vi "FIR_5decimate_5cycles.vi"(7 "reset":bool, 8 "valid in":bool, 10 "Q in":fxp<+/-,16,14>, 11 "I in":fxp<+/-,16,14>) -> (0 "valid out":bool, 2 "Q out":fxp<+/-,16,14>, 3 "I out":fxp<+/-,16,14>, 4 "ready for input":bool)   [LabVIEW 2013]
uses:
  <vilib>/rvi/IPIntegrationNode/IPINode_Utilities/niFpgaIPINodeSimCore.vi
  <vilib>/rvi/XilinxIP/XIPIN_XNode/niFpgaXIPIN.xnode
  Filters/FIR_5decimate_5cycles/FIR_5Decimate_5Cycles_B5291933BF2B454885F1E12D573C96C6.dll
  <vilib>/rvi/IPIntegrationNode/IPINode_Xnode/niFpgaIPINode.xnode
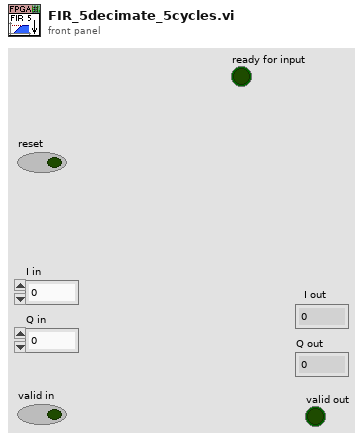
[diagram p1: front panel]
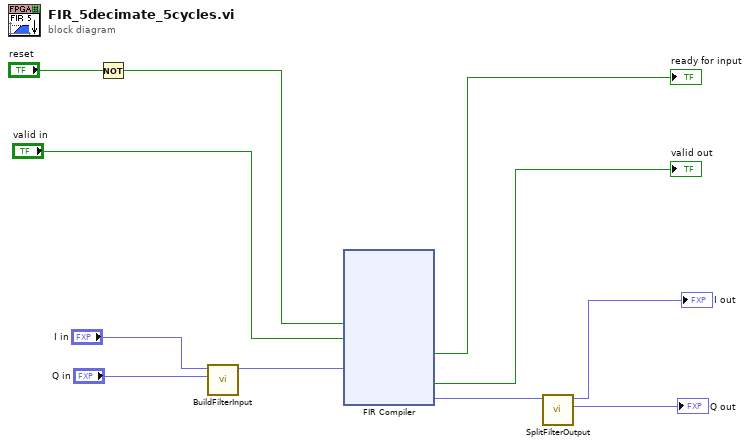
[diagram p0: block diagram]
diagram:
  n1 = Not(x="reset") -> (.not. x?=w10:bool)
  n2 = call "BuildFilterInput.vi"("Q in"="Q in", "I in"="I in") -> ("Filter input"=w6:fxp<+,32,32>)  [unwired: 9 in]
  n3 = xnode ("FIR Compiler")("aresetn"=w10, "s_axis_data_tvalid"="valid in", "s_axis_data_tdata"=w6) -> ("s_axis_data_tready"=→"ready for input":bool, "m_axis_data_tvalid"=→"valid out":bool, "m_axis_data_tdata"=w3:fxp<+,64,64>)  [unwired: 1 in]
  n4 = call "SplitFilterOutput.vi"("filter output"=w3) -> ("Q out"=→"Q out":fxp<+/-,16,14>, "I out"=→"I out":fxp<+/-,16,14>)  [unwired: 9 in]
